vi "Hitrap_DiagnosticBox.ProcCases.vi"(0 "i ref in":refnum<vi>, 1 "selector":string, 2 "Data":T1, 3 "call cluster":T2={"Object"="", "Selector"="", "CallType"=enum."synchronous", "Async Object"="", "Async Selector"="", "Data Descriptor"="", "Data"=[], "Error #"=0, "Expire"=0}, 5 "error in (no error)":errorcluster) -> (14 "i ref out":refnum<vi>, 17 "answer cluster":T2={"Object"="", "Selector"="", "CallType"=enum."synchronous", "Async Object"="", "Async Selector"="", "Data Descriptor"="", "Data"=[], "Error #"=0, "Expire"=0}, 19 "error out":errorcluster)   [LabVIEW 2014, in "Hitrap_DiagnosticBox.lvlib"]
doc: "This method is called by a process from within the default case in the event loop. The methods of a class that are linked to events will be called from THIS method. Add your code here."
uses:
  Hitrap_DiagnosticBox.lvlib
  CSCore/CSSystem/CoreDefs/CoreDefs.call_type.ctl
  CSCore/BaseProcess/BaseProcess.descriptor string definition.ctl
  CSCore/CSSystem/CoreDefs/CoreDefs.rawDataType.ctl
  CSCore/CSSystem/CoreLib/CoreLib.string 2 byte array.vi
  CSCore/CSSystem/CoreLib/CoreLib.double 2 byte array.vi
  CSCore/CSSystem/CoreLib/CoreLib.byte array 2 double.vi
  CSCore/CSSystem/CoreLib/CoreLib.byte array 2 int.vi
  CSCore/CSSystem/CoreLib/CoreLib.lvlib
  CSCore/BaseProcess/BaseProcess.lvlib
  CSMotion/NanotecSMCPD/NanotecSMCPD.lvlib
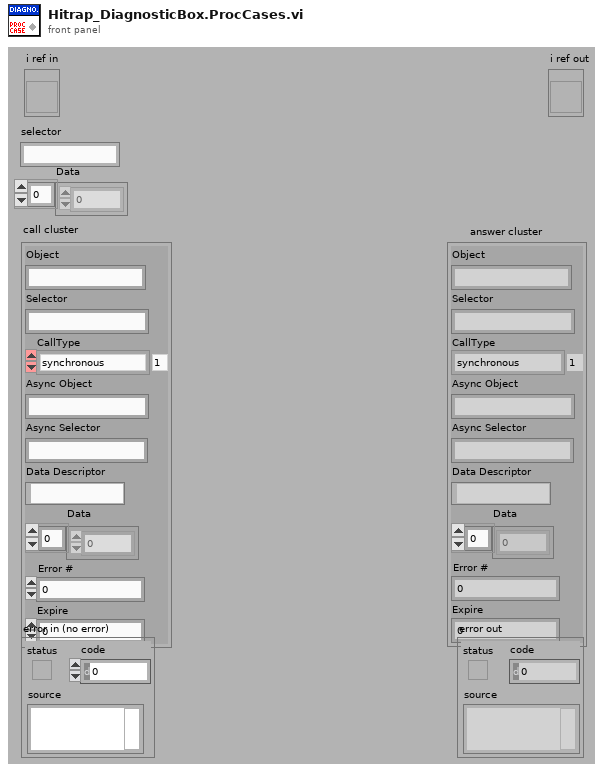
[diagram p1: front panel]
types:
  T1 = typedef "CoreDefs.rawDataType.ctl" = i8[]
  T2 = typedef "CoreDefs.call_type.ctl" = cluster{"Object":string, "Selector":string, "CallType":enum16{"simple", "synchronous", "asynchronous"}, "Async Object":string, "Async Selector":string, "Data Descriptor":T3, "Data":T1, "Error #":i32, "Expire":u32}
  T3 = typedef "BaseProcess.lvlib/BaseProcess.descriptor string definition.ctl" = string
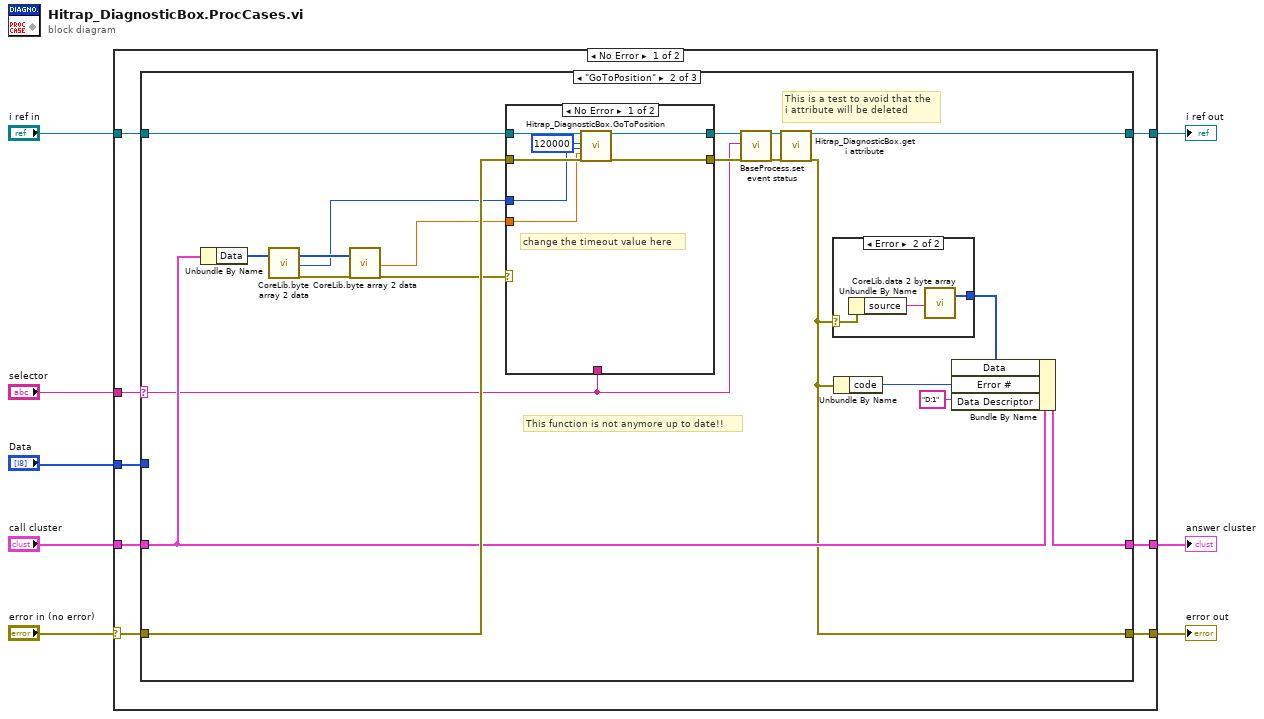
[diagram p0: block diagram]
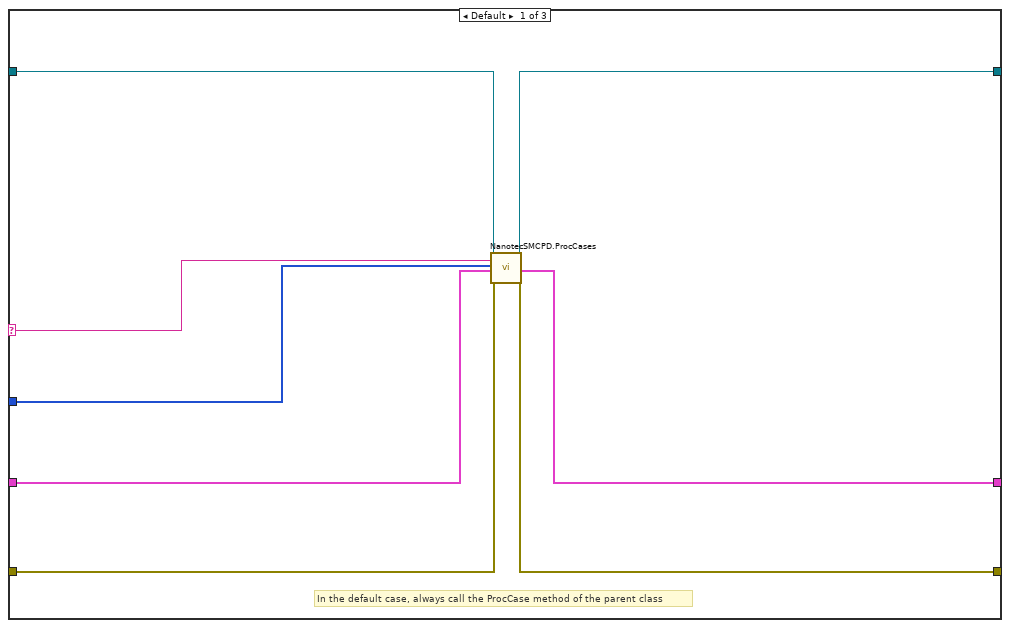
[diagram p2: hidden frame]
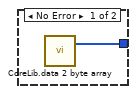
[diagram p3: hidden frame]
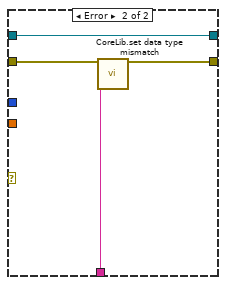
[diagram p4: hidden frame]
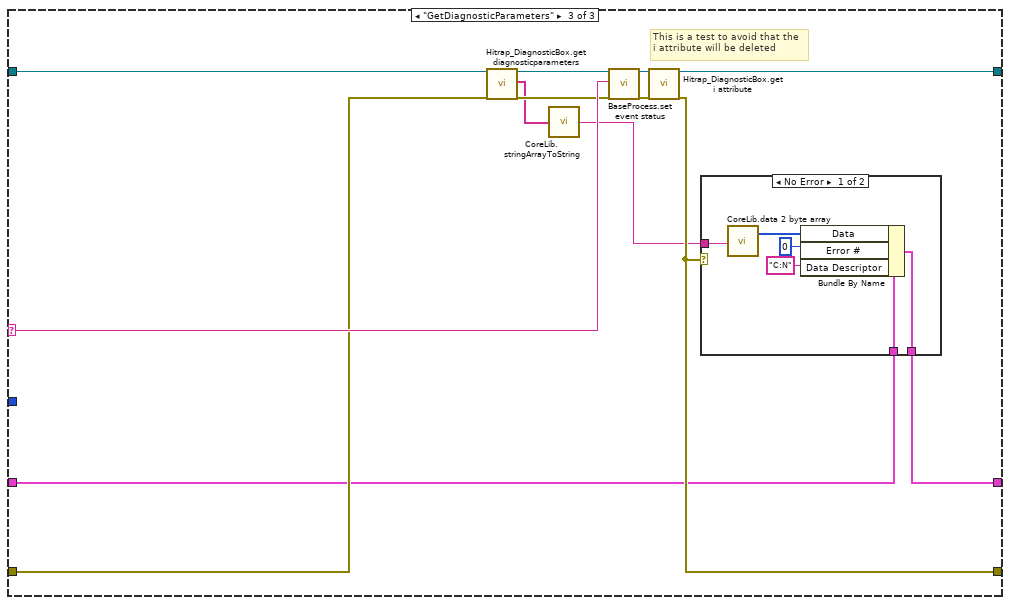
[diagram p5: hidden frame]
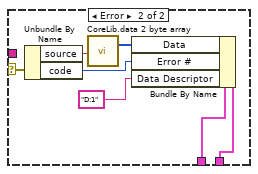
[diagram p6: hidden frame]
diagram:
  n1 = case shown="No Error" "error in (no error)" {
    selector: "error in (no error)" -> [w9 w86]
    tunnel: "selector" -> [w16 _]
    tunnel: [w15 w87] -> w7
    tunnel: "Data" -> [w14 _]
    tunnel: "call cluster" -> [w13 w87]
    tunnel: "i ref in" -> [w12 w88]
    tunnel: [w11 w88] -> w3
    tunnel: [w10 w86] -> w2
    frame No Error {
      n2 = case shown="\"GoToPosition\"" w16 {
        selector: w16 -> [w19 w36 w72]
        tunnel: w14 -> [w17 _ _]
        tunnel: w12 -> [w18 w44 w67]
        tunnel: [w24 w25 w68] -> w11
        tunnel: w13 -> [w20 w41 w61]
        tunnel: [w21 w40 w60] -> w15
        tunnel: w9 -> [w23 w43 w64]
        tunnel: [w22 w27 w70] -> w10
        frame Default {
          # "In the default case, always call the ProcCase method of the parent class"
          n3 = call "NanotecSMCPD.ProcCases.vi"("i ref in"=w18, "selector"=w19, "Data"=w17, "call cluster"=w20, "error in (no error)"=w23) -> ("i ref out"=w24:refnum<vi>, "answer cluster"=w21:T2, "error out"=w22:errorcluster)  [unwired: 12 in]
        }
        frame "GoToPosition" {
          # "This function is not anymore up to date!!"
          # "This is a test to avoid that the\ni attribute will be deleted"
          n4 = Unbundle By Name(w41) -> ("Data"=w34:T1)
          n5 = call-poly "CoreLib.byte array 2 data.vi"("byteArray"=w34) -> ("byteArray out"=w33:T1, "i32"=w31:i32, "error out"=w32:errorcluster)  [unwired: 16 in]
          n6 = call-poly "CoreLib.byte array 2 data.vi"("byteArray"=w33, "error in (no error)"=w32) -> ("d64"=w30:dbl, "error out"=w29:errorcluster)  [unwired: 15 in, 1 out]
          n7 = case shown="No Error" w29 {
            tunnel: [w53 w59] -> w38
            tunnel: w44 -> [w54 w59]
            tunnel: w43 -> [w55 w58]
            tunnel: [w52 w57] -> w37
            tunnel: w30 -> [w51 _]
            tunnel: w36 -> [_ w56]
            tunnel: w31 -> [w50 _]
            frame No Error {
              # "change the timeout value here"
              n8 = call "Hitrap_DiagnosticBox.GoToPosition.vi"("i ref in"=w54, "Timeout"=120000, "Axis"=w50, "StepsFromPosition"=w51, "error in"=w55) -> ("i ref out"=w53:refnum<vi>, "error out"=w52:errorcluster)  [unwired: 13 in]
            }
            frame Error {
              n9 = call "CoreLib.set data type mismatch.vi"("error in (no error)"=w58, "error source"=w56) -> ("error out"=w57:errorcluster)  [unwired: 17 in]
            }
          }
          n10 = call "BaseProcess.set event status.vi"("i ref in"=w38, "EventStatus"=w36, "error in (no error)"=w37) -> ("i ref out"=w26:refnum<vi>, "error out"=w28:errorcluster)  [unwired: 14 in, 1 out]
          n11 = call "Hitrap_DiagnosticBox.get i attribute.vi"("i ref in"=w26, "error in (no error)"=w28) -> ("i ref out"=w25:refnum<vi>, "error out"=w27:errorcluster)  [unwired: 15 in, 1 out]
          n12 = case shown="Error" w27 {
            selector: w27 -> [_ w48]
            tunnel: [w45 w47] -> w39
            frame No Error {
              n13 = call-poly "CoreLib.data 2 byte array.vi"() -> ("byteArray out"=w45:T1)  [unwired: 19 in]
            }
            frame Error {
              n14 = Unbundle By Name(w48) -> ("source"=w46:string)
              n15 = call-poly "CoreLib.data 2 byte array.vi"("string"=w46) -> ("byteArray out"=w47:T1)  [unwired: 18 in]
            }
          }
          n16 = Unbundle By Name(w27) -> ("code"=w42:i32)
          n17 = Bundle By Name(cluster=w41, "Data"=w39, "Error #"=w42, "Data Descriptor"="D:1") -> (w40:T2)
        }
        frame "GetDiagnosticParameters" {
          # "This is a test to avoid that the\ni attribute will be deleted"
          n18 = call "Hitrap_DiagnosticBox.get diagnosticparameters.vi"("i ref in"=w67, "error in (no error)"=w64) -> ("i ref out"=w66:refnum<vi>, "appended array"=w63:string[], "error out"=w65:errorcluster)  [unwired: 15 in]
          n19 = call "CoreLib.stringArrayToString.vi"("Array"=w63) -> ("String"=w62:string)
          n20 = call "BaseProcess.set event status.vi"("i ref in"=w66, "EventStatus"=w72, "error in (no error)"=w65) -> ("i ref out"=w69:refnum<vi>, "error out"=w71:errorcluster)  [unwired: 14 in, 1 out]
          n21 = call "Hitrap_DiagnosticBox.get i attribute.vi"("i ref in"=w69, "error in (no error)"=w71) -> ("i ref out"=w68:refnum<vi>, "error out"=w70:errorcluster)  [unwired: 15 in, 1 out]
          n22 = case shown="No Error" w70 {
            selector: w70 -> [_ w85]
            tunnel: w62 -> [w78 _]
            tunnel: w61 -> [w75 w83]
            tunnel: [w74 w82] -> w60
            frame No Error {
              n23 = call-poly "CoreLib.data 2 byte array.vi"("string"=w78) -> ("byteArray out"=w76:T1)  [unwired: 18 in]
              n24 = Bundle By Name(cluster=w75, "Data"=w76, "Error #"=0, "Data Descriptor"="C:N") -> (w74:T2)
            }
            frame Error {
              n25 = Unbundle By Name(w85) -> ("source"=w84:string, "code"=w80:i32)
              n26 = call-poly "CoreLib.data 2 byte array.vi"("string"=w84) -> ("byteArray out"=w81:T1)  [unwired: 18 in]
              n27 = Bundle By Name(cluster=w83, "Data"=w81, "Error #"=w80, "Data Descriptor"="D:1") -> (w82:T2)
            }
          }
        }
      }
    }
    frame Error {
    }
  }
  "answer cluster" <- w7
  "i ref out" <- w3
  "error out" <- w2
